vi "http.post_binary.vi"(6 "specific headers in":cluster{"header":string, "Value":string}[](array[cluster]), 7 "Content Type":string="application/json", 8 "error in":errorcluster, 9 "Request body":string, 10 "Path":string, 11 "Nominal Client in":refnum<class "Nominal Client.lvclass">) -> (0 "error out":errorcluster, 2 "Response":string, 3 "Nominal Client out":refnum<class "Nominal Client.lvclass">)   [LabVIEW 2020, in "Nominal Client.lvclass"]
uses:
  Nominal Client.lvclass
  Nominal Client.lvclass/Nominal Client.ctl
  <vilib>/addons/_JKI.lib/REST Client/classes/REST Client/REST Client.lvclass
  reqwest/reQwestClient.lvclass
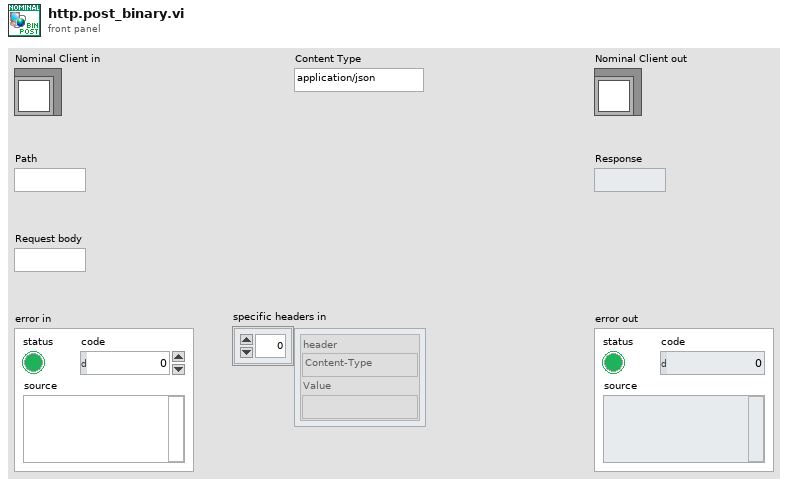
[diagram p1: front panel]
types:
  T1 = typedef "Nominal Client.lvclass/private_data.ctl" = cluster{"API Token":string, "workspace":refnum<class "workspace.lvclass">, "Available Workspaces":refnum<class "workspace.lvclass">[], "REST Client":cluster{"Client":enum16{"JKI HTTP REST", "reQwest"}, "HTTP REST":refnum<class "REST Client.lvclass">, "reQwest":refnum<class "reQwestClient.lvclass">}}
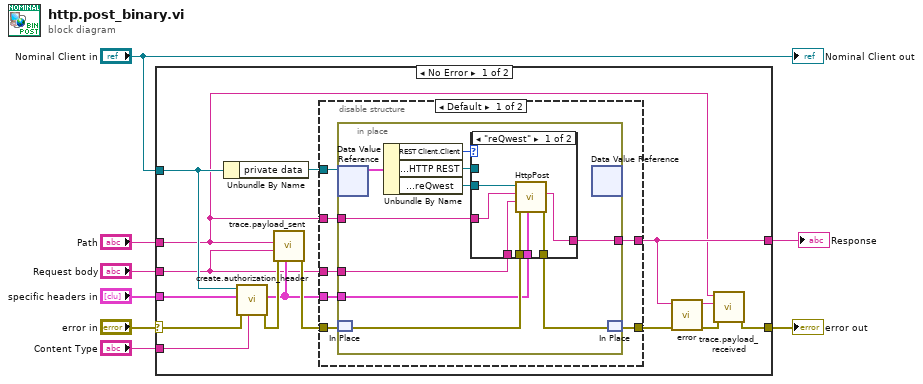
[diagram p0: block diagram]
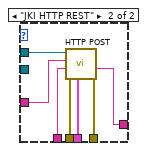
[diagram p2: hidden frame]
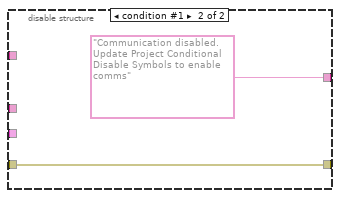
[diagram p3: hidden frame]
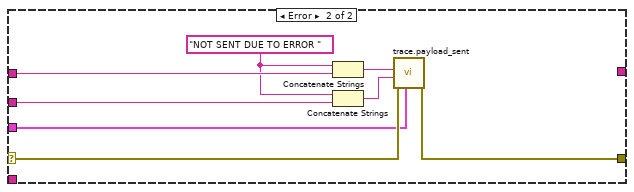
[diagram p4: hidden frame]
diagram:
  n1 = case shown="No Error" "error in" {
    selector: "error in" -> [w17 w59]
    tunnel: "Nominal Client in" -> [w21 _]
    tunnel: "specific headers in" -> [w18 w57]
    tunnel: "Request body" -> [w16 w61]
    tunnel: "Content Type" -> [w15 _]
    tunnel: [w14 _] -> w3
    tunnel: [w9 w58] -> w2
    tunnel: "Path" -> [w11 w63]
    frame No Error {
      n2 = Unbundle By Name(w21) -> ("private data"=w19:refnum<data-value>)
      n3 = call "create.authorization_header.vi"("Content Type"=w15, "error in"=w17, "specific headers in"=w18, "Nominal Client in"=w21) -> ("error out"=w23:errorcluster, "specific headers out"=w20:cluster{"header":string, "value":string}[])  [unwired: 5 in, 1 out]
      n4 = call "trace.payload_sent.vi"("Headers"=w20, "dataflow error in"=w23, "Request Body"=w16, "Path"=w11) -> ("dataflow error out"=w22:errorcluster)  [unwired: 7 in]
      n5 = disable-structure shown="Default" {
        disable-tunnel: w20 -> [w30 _]
        disable-tunnel: w19 -> [w29 _]
        disable-tunnel: w22 -> [w28 w56]
        disable-tunnel: w16 -> [w27 _]
        disable-tunnel: [w26 "Communication disabled. Update Project Conditional Disable Symbols to enable comms" ("REST Response")] -> w14
        disable-tunnel: [w25 w56] -> w12
        disable-tunnel: w11 -> [w24 _]
        frame condition #0 (active) {
          n6 = in-place {
            in-place-border: w30 -> [w36]
            in-place-border: [w38] -> w26
            in-place-border: w24 -> [w35]
            in-place-border: w27 -> [w37]
            n7 = in-place-dvr #1(w29) -> (w40:T1)  [unwired: 1 out]
            n8 = in-place-match #2(w28) -> (w39:errorcluster)
            n9 = Unbundle By Name(w40) -> ("REST Client.Client"=w33:enum16{"JKI HTTP REST", "reQwest"}, "REST Client.HTTP REST"=w32:refnum<class "REST Client.lvclass">, "REST Client.reQwest"=w31:refnum<class "reQwestClient.lvclass">)
            n10 = case shown="\"reQwest\"" w33 {
              tunnel: w39 -> [w41 w54]
              tunnel: [w42 w53] -> w38
              tunnel: w37 -> [w45 w52]
              tunnel: w36 -> [w44 w51]
              tunnel: w35 -> [w46 w50]
              tunnel: [w43 w49] -> w34
              tunnel: w32 -> [_ w48]
              tunnel: w31 -> [w47 _]
              frame "reQwest" {
                n11 = call "HttpPost.vi"("request specific headers"=w44, "error in"=w41, "body"=w45, "url"=w46, "reQwestClient in"=w47) -> ("error out"=w43:errorcluster, "response_body"=w42:string)  [unwired: 3 in, 2 out]
              }
              frame "JKI HTTP REST" {
                n12 = call-dynamic "HTTP POST.vi"("request specific headers"=w51, "error in (no error)"=w54, "Request body"=w52, "Path"=w50, "REST Client in"=w48) -> ("error out"=w49:errorcluster, "Response body"=w53:string)  [unwired: 1 in, 4 out]
              }
            }
            n13 = in-place-dvr #1() -> ()  [unwired: 1 in, 2 out]
            n14 = in-place-match #2(w34) -> (w25:errorcluster)
          }
        }
        frame condition #1 {
        }
      }
      n15 = call "error.vi"("error in"=w12, "REST Response"=w14) -> ("error out"=w10:errorcluster, "Error Formatted Response"=w13:string)  [unwired: 8 in]
      n16 = call "trace.payload_received.vi"("dataflow error in"=w10, "Response"=w13, "Path"=w11) -> ("dataflow error out"=w9:errorcluster)  [unwired: 8 in]
    }
    frame Error {
      w62 = "NOT SENT DUE TO ERROR " ("string")
      n17 = Concatenate Strings(w62, w63) -> (w64:string)
      n18 = Concatenate Strings(w62, w61) -> (w60:string)
      n19 = call "trace.payload_sent.vi"("Headers"=w57, "dataflow error in"=w59, "Request Body"=w60, "Path"=w64) -> ("dataflow error out"=w58:errorcluster)  [unwired: 7 in]
    }
  }
  "error out" <- w2
  "Response" <- w3
  "Nominal Client out" <- "Nominal Client in"
